vi "Client_Template_MOD.vi"() -> ()   [LabVIEW 2025]
panel:
  in  "Logging?":bool
  in  "Logging File Name":string="Default_Log_Name"
  in  "Enable \nExternal \nCommunication":bool
  out "Scratch Output 7":dbl
  out "Scratch Output 6":dbl
  out "Scratch Output 5":dbl
  out "Scratch Output 4":dbl
  out "Scratch Output 3":dbl
  out "Scratch Output 2":dbl
  out "Scratch Output 1":dbl
  out "Scratch Output 0":dbl
  out "Scratch Input 7":dbl
  out "Scratch Input 6":dbl
  out "Scratch Input 5":dbl
  out "Scratch Input 4":dbl
  out "Scratch Input 3":dbl
  out "Scratch Input 2":dbl
  out "Scratch Input 1":dbl
  out "Scratch Input 0":dbl
  out "Iteration#":i32=11
  out "Status Display":errorcluster={"status"=FALSE, "code"=0, "source"="Post passed -- System successfully initialised"}
  out "t (sec)":dbl=4.42
  out "Loop Status":bool=TRUE
  in  "dt (ms)":u32=200
  in  "ES#":T1(ring)
  in  "stop":bool
  in  "DI:CH0":T2(ring)
  in  "DO:CH0":T3(ring)
  in  "AO:CH1":T4(ring)=enum."AO-1"
  in  "AO:CH0":T4(ring)
  in  "Analog Output 2":dbl(slide) scale=0.0..100.0
  in  "Analog Output 1":dbl(slide) scale=0.0..100.0
  out "Analog Input 2":dbl(slide)=50.0 scale=0.0..100.0
  in  "AI:CH1":T5(ring)=enum."AI-1"
  in  "AI:CH0":T5(ring)
  out "Digital Input":bool
  in  "Digital Output":bool
  out "Analog Input 1":dbl(slide)=50.0 scale=0.0..100.0
  out "Waveform Chart":T6(graph)={"Analog Input 1"=50.0, "Analog Input 1"=50.0, "Analog Output 1"=0.0, "Analog Output 2"=0.0}
  # "Data Logging: \nAll files saved as .csv format to:\nproject file -> Labview_Logging"
  # "FROM EXTERNAL:"
  # "TO EXTERNAL:"
  # "Experimental Template"
  # "Basic Experimental Template"
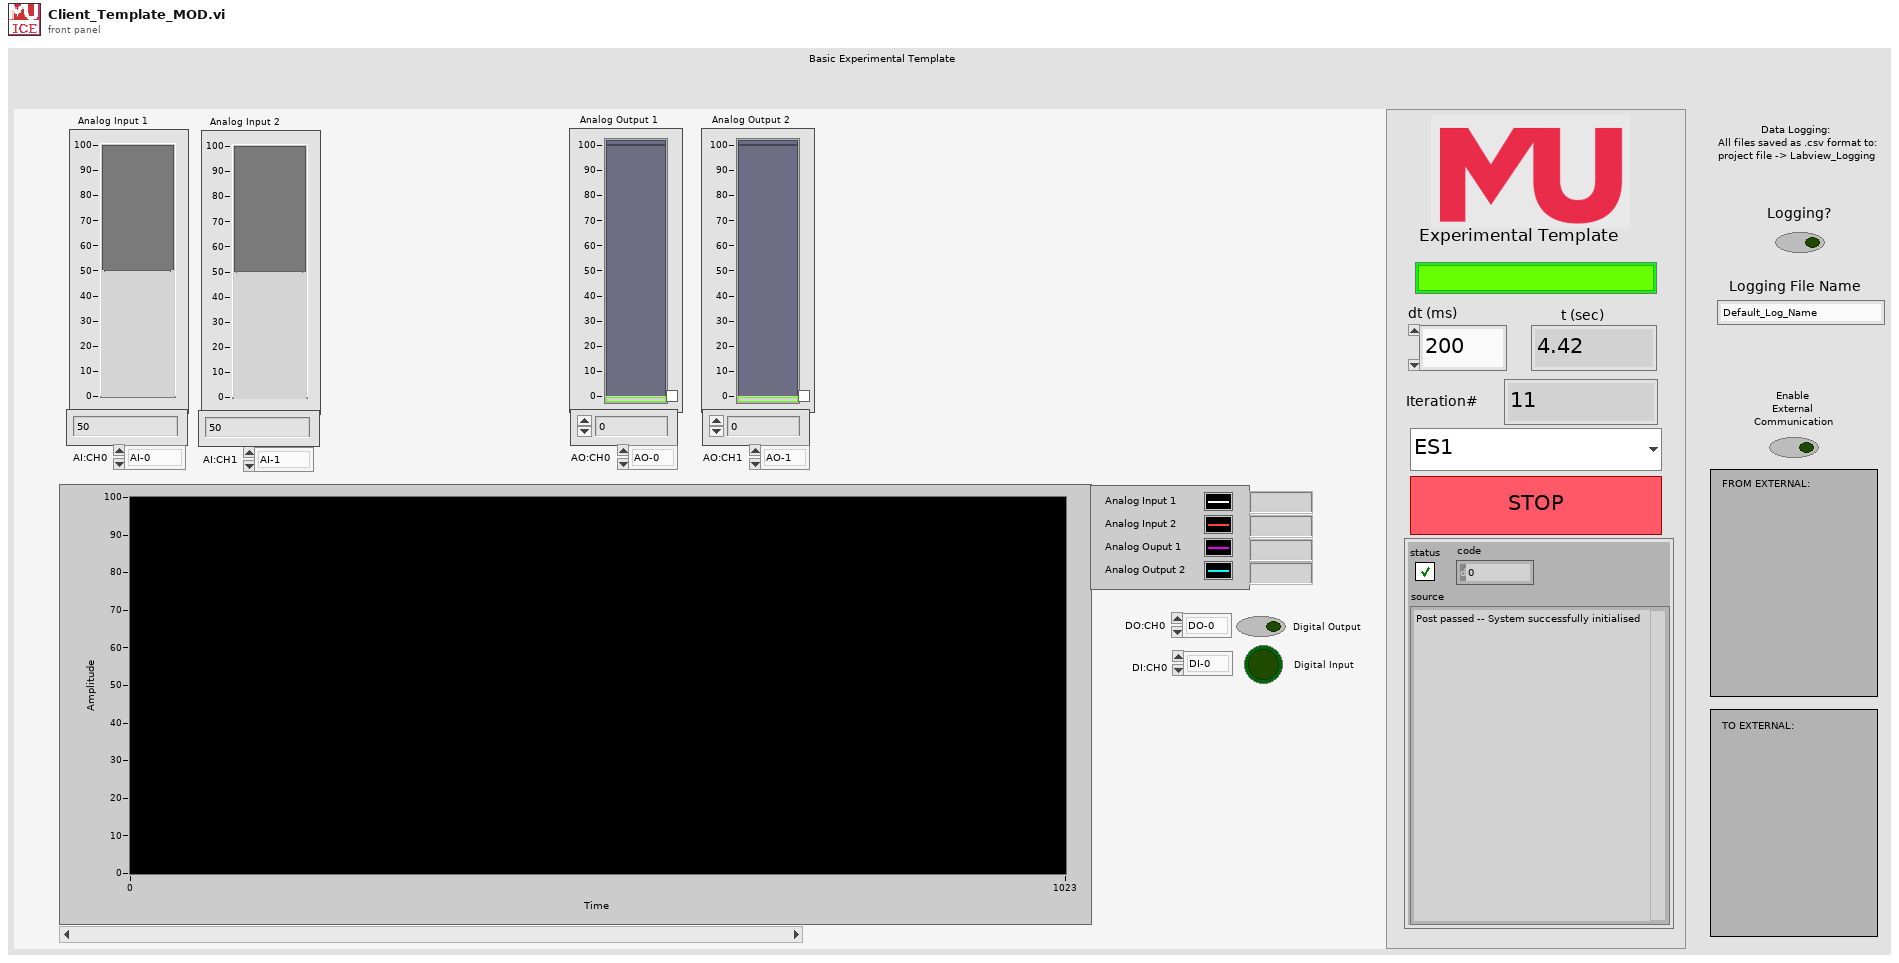
[diagram p1: front panel]
types:
  T1 = enum16{"ES1", "ES2", "ES3", "ES4", "ES5", "ES6", "ES7", "ES8"}
  T2 = enum16{"DI-0", "DI-1", "DI-2", "DI-3", "DI-4", "DI-5", "DI-6", "DI-7"}
  T3 = enum16{"DO-0", "DO-1", "DO-2", "DO-3", "DO-4", "DO-5", "DO-6", "DO-7"}
  T4 = enum16{"AO-0", "AO-1", "AO-2", "AO-3", "AO-4", "AO-5", "AO-6", "AO-7"}
  T5 = enum16{"AI-0", "AI-1", "AI-2", "AI-3", "AI-4", "AI-5", "AI-6", "AI-7"}
  T6 = cluster{"Analog Input 1":dbl, "Analog Input 1":dbl, "Analog Output 1":dbl, "Analog Output 2":dbl}
  T7 = cluster{u16, u32, "Modbus master out":refnum<class "Modbus Master.lvclass">}
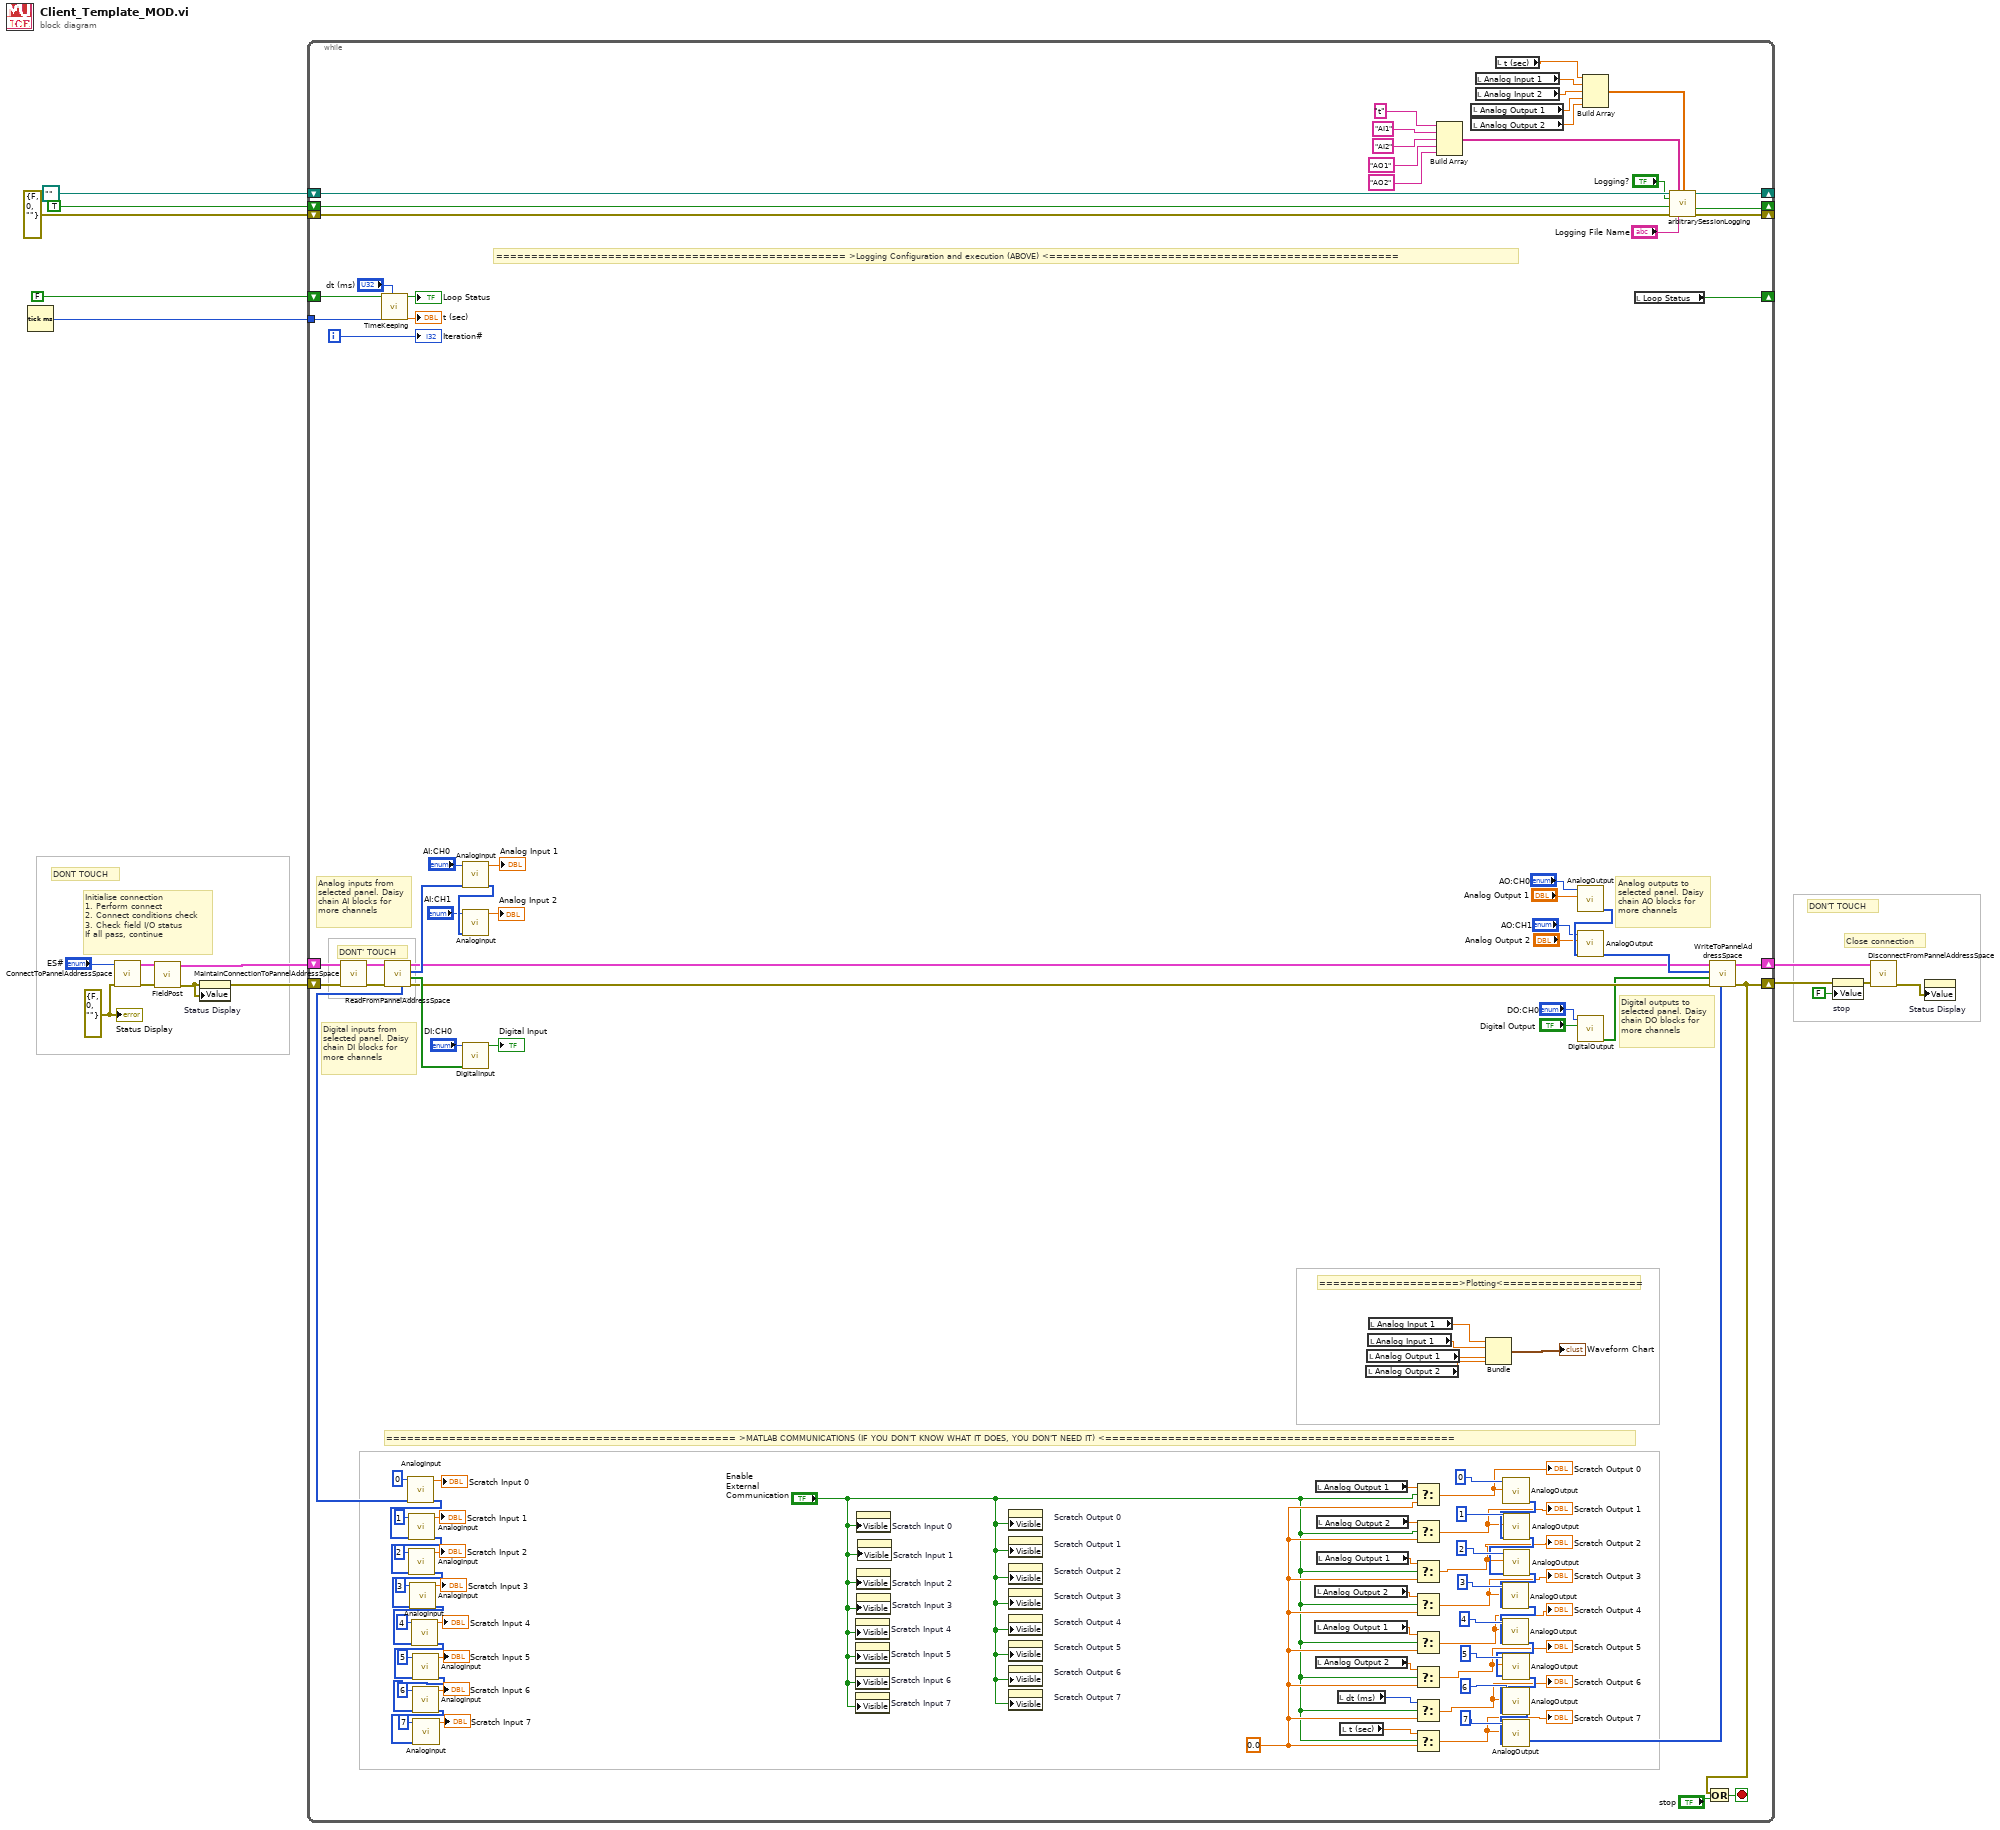
[diagram p0: block diagram]
diagram:
  w5 = errorcluster {"status"=FALSE, "code"=0, "source"=""} ("error out")
  # "DON'T TOUCH"
  # "DONT TOUCH"
  # "Close connection"
  # "Initialise connection\n1. Perform connect\n2. Connect conditions check\n3. Check field I/O status\nIf all pass, continue"
  n1 = Tick Count (ms)() -> (millisecond timer value=w16:u32)
  n2 = call "ConnectToPannelAddressSpace.vi"("error in (no error)"=w5, "Station#"="ES#") -> ("error out"=w2:errorcluster, "comms cluster"=w1:T7)  [unwired: 6 in, 2 out]
  n3 = call "FieldPost.vi"("error in (no error)"=w2, "comms cluster in"=w1) -> ("error out"=w3:errorcluster, "comms cluster out"=w7:T7)  [unwired: 8 in]
  n4 = property on="Status Display" class="Clust (strict)"(error in=w3, "Value"=w3) -> (error out=w6:errorcluster)  [unwired: 1 in, 1 out]
  n5 = while {
    shift-right: [w20] -> w17
    shift-left: w7 -> [w19]
    shift-right: [w21] -> w9
    shift-left: w6 -> [w18]
    tunnel: w16 -> [w48]
    shift-right: [w117] -> _
    shift-left: FALSE -> [w128]
    shift-right: [w35] -> _
    shift-left: path "" ("new file path (Not A Path if cancelled)") -> [w34]
    shift-right: [w36] -> _
    shift-left: errorcluster {"status"=FALSE, "code"=0, "source"=""} ("error out") -> [w37]
    shift-right: [w23] -> _
    shift-left: TRUE -> [w32]
    i -> [w109]
    stop <- w135 stop-if-true
    w53 = 0.0 ("f")
    # "DONT' TOUCH"
    # "================================================== >Logging Configuration and execution (ABOVE) <=================================================="
    # "Digital outputs to\nselected panel. Daisy\nchain DO blocks for\nmore channels"
    # "Digital inputs from\nselected panel. Daisy\nchain DI blocks for\nmore channels"
    # "Analog outputs to\nselected panel. Daisy\nchain AO blocks for\nmore channels"
    # "Analog inputs from\nselected panel. Daisy\nchain AI blocks for\nmore channels"
    # "================================================== >MATLAB COMMUNICATIONS (IF YOU DON'T KNOW WHAT IT DOES, YOU DON'T NEED IT) <=================================================="
    # "====================>Plotting<===================="
    n6 = call "MaintainConnectionToPannelAddressSpace.vi"("error in (no error)"=w18, "comms cluster in"=w19) -> ("error out"=w133:errorcluster, "comms cluster out"=w134:T7)  [unwired: 7 in, 1 out]
    n7 = call "TimeKeeping.vi"("dt desired (ms)"="dt (ms)", "start tick"=w48, "Prev Loop Status"=w128) -> ("time since start (s)"=→"t (sec)":dbl, "Current Loop Status"=→"Loop Status":bool)  [unwired: 7 in]
    n8 = call "ReadFromPannelAddressSpace.vi"("error in (no error)"=w133, "comms cluster in"=w134) -> ("error out"=w130:errorcluster, "input discrete"=w131:bool[], "input registers"=w132:u16[], "comms cluster out"=w44:T7, "scratch input registers"=w108:u16[])  [unwired: 5 in]
    n9 = call "AnalogInput.vi"("Analog Input Channel"=0, "register values IN"=w108) -> ("Analog Value"=→"Scratch Input 0":dbl, "register values OUT"=w92:u16[])  [unwired: 7 in]
    n10 = call "AnalogInput.vi"("Analog Input Channel"=1, "register values IN"=w92) -> ("Analog Value"=→"Scratch Input 1":dbl, "register values OUT"=w91:u16[])  [unwired: 7 in]
    n11 = call "AnalogInput.vi"("Analog Input Channel"=2, "register values IN"=w91) -> ("Analog Value"=→"Scratch Input 2":dbl, "register values OUT"=w90:u16[])  [unwired: 7 in]
    n12 = call "AnalogInput.vi"("Analog Input Channel"=3, "register values IN"=w90) -> ("Analog Value"=→"Scratch Input 3":dbl, "register values OUT"=w89:u16[])  [unwired: 7 in]
    n13 = call "AnalogInput.vi"("Analog Input Channel"=4, "register values IN"=w89) -> ("Analog Value"=→"Scratch Input 4":dbl, "register values OUT"=w88:u16[])  [unwired: 7 in]
    n14 = call "AnalogInput.vi"("Analog Input Channel"=5, "register values IN"=w88) -> ("Analog Value"=→"Scratch Input 5":dbl, "register values OUT"=w87:u16[])  [unwired: 7 in]
    n15 = call "AnalogInput.vi"("Analog Input Channel"=6, "register values IN"=w87) -> ("Analog Value"=→"Scratch Input 6":dbl, "register values OUT"=w86:u16[])  [unwired: 7 in]
    n16 = call "AnalogInput.vi"("Analog Input Channel"=7, "register values IN"=w86) -> ("Analog Value"=→"Scratch Input 7":dbl)  [unwired: 7 in, 1 out]
    n17 = call "AnalogInput.vi"("Analog Input Channel"="AI:CH0", "register values IN"=w132) -> ("Analog Value"=→"Analog Input 1":dbl, "register values OUT"=w127:u16[])  [unwired: 7 in]
    n18 = call "AnalogInput.vi"("Analog Input Channel"="AI:CH1", "register values IN"=w127) -> ("Analog Value"=→"Analog Input 2":dbl)  [unwired: 7 in, 1 out]
    n19 = call "DigitalInput.vi"("discrete input values IN"=w131, "Digital Input Channel"="DI:CH0") -> ("Digital Value"=→"Digital Input":bool)  [unwired: 8 in, 1 out]
    n20 = property on="Scratch Input 4" class="DigNum (strict)"("Visible"="Enable \nExternal \nCommunication") -> ()  [unwired: 2 in, 2 out]
    n21 = property on="Scratch Input 5" class="DigNum (strict)"("Visible"="Enable \nExternal \nCommunication") -> ()  [unwired: 2 in, 2 out]
    n22 = property on="Scratch Input 6" class="DigNum (strict)"("Visible"="Enable \nExternal \nCommunication") -> ()  [unwired: 2 in, 2 out]
    n23 = property on="Scratch Input 7" class="DigNum (strict)"("Visible"="Enable \nExternal \nCommunication") -> ()  [unwired: 2 in, 2 out]
    n24 = property on="Scratch Input 0" class="DigNum (strict)"("Visible"="Enable \nExternal \nCommunication") -> ()  [unwired: 2 in, 2 out]
    n25 = property on="Scratch Input 2" class="DigNum (strict)"("Visible"="Enable \nExternal \nCommunication") -> ()  [unwired: 2 in, 2 out]
    n26 = property on="Scratch Input 3" class="DigNum (strict)"("Visible"="Enable \nExternal \nCommunication") -> ()  [unwired: 2 in, 2 out]
    n27 = property on="Scratch Input 1" class="DigNum (strict)"("Visible"="Enable \nExternal \nCommunication") -> ()  [unwired: 2 in, 2 out]
    n28 = property on="Scratch Output 0" class="DigNum (strict)"("Visible"="Enable \nExternal \nCommunication") -> ()  [unwired: 2 in, 2 out]
    n29 = property on="Scratch Output 1" class="DigNum (strict)"("Visible"="Enable \nExternal \nCommunication") -> ()  [unwired: 2 in, 2 out]
    n30 = property on="Scratch Output 2" class="DigNum (strict)"("Visible"="Enable \nExternal \nCommunication") -> ()  [unwired: 2 in, 2 out]
    n31 = property on="Scratch Output 3" class="DigNum (strict)"("Visible"="Enable \nExternal \nCommunication") -> ()  [unwired: 2 in, 2 out]
    n32 = property on="Scratch Output 4" class="DigNum (strict)"("Visible"="Enable \nExternal \nCommunication") -> ()  [unwired: 2 in, 2 out]
    n33 = property on="Scratch Output 5" class="DigNum (strict)"("Visible"="Enable \nExternal \nCommunication") -> ()  [unwired: 2 in, 2 out]
    n34 = property on="Scratch Output 6" class="DigNum (strict)"("Visible"="Enable \nExternal \nCommunication") -> ()  [unwired: 2 in, 2 out]
    n35 = property on="Scratch Output 7" class="DigNum (strict)"("Visible"="Enable \nExternal \nCommunication") -> ()  [unwired: 2 in, 2 out]
    n36 = local read "Analog Output 2"() -> (w63:dbl)
    n37 = local read "Analog Output 1"() -> (w61:dbl)
    n38 = local read "Analog Output 1"() -> (w69:dbl)
    n39 = local read "Analog Output 2"() -> (w59:dbl)
    n40 = local read "Analog Output 2"() -> (w67:dbl)
    n41 = local read "Analog Output 1"() -> (w65:dbl)
    n42 = local read "dt (ms)"() -> (w57:u32)
    n43 = local read "t (sec)"() -> (w55:dbl)
    n44 = local read "Analog Output 2"() -> (w22:dbl)
    n45 = local read "Analog Output 1"() -> (w118:dbl)
    n46 = local read "Analog Input 1"() -> (w119:dbl)
    n47 = local read "Analog Input 1"() -> (w120:dbl)
    n48 = Select(t=w69, s="Enable \nExternal \nCommunication", f=w53) -> (s? t:f=w68:dbl)
    "Scratch Output 0" <- w68
    n49 = Select(t=w67, s="Enable \nExternal \nCommunication", f=w53) -> (s? t:f=w66:dbl)
    "Scratch Output 1" <- w66
    n50 = Select(t=w65, s="Enable \nExternal \nCommunication", f=w53) -> (s? t:f=w64:dbl)
    "Scratch Output 2" <- w64
    n51 = Select(t=w63, s="Enable \nExternal \nCommunication", f=w53) -> (s? t:f=w62:dbl)
    "Scratch Output 3" <- w62
    n52 = Select(t=w61, s="Enable \nExternal \nCommunication", f=w53) -> (s? t:f=w60:dbl)
    "Scratch Output 4" <- w60
    n53 = Select(t=w59, s="Enable \nExternal \nCommunication", f=w53) -> (s? t:f=w58:dbl)
    "Scratch Output 5" <- w58
    n54 = Select(t=w57, s="Enable \nExternal \nCommunication", f=w53) -> (s? t:f=w56:dbl)
    "Scratch Output 6" <- w56
    n55 = Select(t=w55, s="Enable \nExternal \nCommunication", f=w53) -> (s? t:f=w54:dbl)
    "Scratch Output 7" <- w54
    n56 = Build Array("t" ("delimiter (\\t)"), "AI1" ("delimiter (\\t)"), "AI2" ("delimiter (\\t)"), "AO1" ("delimiter (\\t)"), "AO2" ("delimiter (\\t)")) -> (w30:string[])
    n57 = local read "Analog Output 1"() -> (w25:dbl)
    n58 = local read "Analog Output 2"() -> (w24:dbl)
    n59 = local read "Analog Input 1"() -> (w27:dbl)
    n60 = local read "Analog Input 2"() -> (w26:dbl)
    n61 = Bundle("Analog Input 1"=w120, "Analog Input 1"=w119, "Analog Output 1"=w118, "Analog Output 2"=w22) -> (→"Waveform Chart":T6)  [unwired: 1 in]
    n62 = local read "t (sec)"() -> (w28:dbl)
    n63 = call "AnalogOutput.vi"("Analog output"=w68, "Output Channel"=0) -> ("Updated output array"=w77:i32[])  [unwired: 9 in]
    n64 = call "AnalogOutput.vi"("Output array"=w77, "Analog output"=w66, "Output Channel"=1) -> ("Updated output array"=w76:i32[])  [unwired: 8 in]
    n65 = call "AnalogOutput.vi"("Output array"=w76, "Analog output"=w64, "Output Channel"=2) -> ("Updated output array"=w75:i32[])  [unwired: 8 in]
    n66 = call "AnalogOutput.vi"("Output array"=w75, "Analog output"=w62, "Output Channel"=3) -> ("Updated output array"=w74:i32[])  [unwired: 8 in]
    n67 = call "AnalogOutput.vi"("Output array"=w74, "Analog output"=w60, "Output Channel"=4) -> ("Updated output array"=w73:i32[])  [unwired: 8 in]
    n68 = call "AnalogOutput.vi"("Output array"=w73, "Analog output"=w58, "Output Channel"=5) -> ("Updated output array"=w72:i32[])  [unwired: 8 in]
    n69 = call "AnalogOutput.vi"("Output array"=w72, "Analog output"=w56, "Output Channel"=6) -> ("Updated output array"=w71:i32[])  [unwired: 8 in]
    n70 = call "AnalogOutput.vi"("Output array"=w71, "Analog output"=w54, "Output Channel"=7) -> ("Updated output array"=w70:i32[])  [unwired: 8 in]
    n71 = call "AnalogOutput.vi"("Analog output"="Analog Output 1", "Output Channel"="AO:CH0") -> ("Updated output array"=w126:i32[])  [unwired: 9 in]
    n72 = call "AnalogOutput.vi"("Output array"=w126, "Analog output"="Analog Output 2", "Output Channel"="AO:CH1") -> ("Updated output array"=w45:i32[])  [unwired: 8 in]
    n73 = call "DigitalOutput.vi"("Digital Output"="Digital Output", "Output Channel"="DO:CH0") -> ("Updated array out"=w129:bool[])  [unwired: 9 in]
    n74 = Build Array(w28, w27, w26, w25, w24) -> (w29:dbl[])
    n75 = local read "Loop Status"() -> (w117:bool)
    n76 = call "arbitrarySessionLogging.vi"("file path in"=w34, "Column Names"=w30, "Log Values"=w29, "Logging?"="Logging?", "Log on previous loop"=w32, "error in (no error)"=w37, "Logging File Name"="Logging File Name") -> ("file path out"=w35:path, "Log for next loop"=w23:bool, "error out"=w36:errorcluster)  [unwired: 6 in]
    n77 = call "WriteToPannelAddressSpace.vi"("Scratch Output Values"=w70, "error in (no error)"=w130, "Digital Write Values"=w129, "Analog Write Values"=w45, "comms cluster in"=w44) -> ("error out"=w21:errorcluster, "comms cluster out"=w20:T7)  [unwired: 5 in]
    n78 = Or(x=w21, y="stop") -> (x .or. y?=w135:bool)
    "Iteration#" <- w109
  }
  n79 = property on="stop" class="Bool (strict)"(error in=w9, "Value"=FALSE ("stop")) -> (error out=w8:errorcluster)  [unwired: 1 in, 1 out]
  n80 = call "DisconnectFromPannelAddressSpace.vi"("error in (no error)"=w8, "comms cluster"=w17) -> ("error out"=w4:errorcluster)  [unwired: 9 in]
  n81 = property on="Status Display" class="Clust (strict)"("Value"=w4) -> ()  [unwired: 2 in, 2 out]
  "Status Display" <- w5
